vi "Read Both Fans Fault and State.vi"(8 "error in (no error)":cluster{"状态":bool, "代码":i32, "源":string} caption="错误输入（无错误）", 11 "双风扇输入":refnum<class "Dual Fan.lvclass">) -> (0 "error out":cluster{"状态":bool, "代码":i32, "源":string} caption="错误输出", 1 "风扇B故障":bool, 2 "风扇B状态":bool, 3 "风扇A故障":bool, 5 "风扇A状态":bool)   [LabVIEW 2015, in "Dual Fan.lvlib" / "Dual Fan.lvclass"]
doc: "子类中必须对该方法进行重写以读取两个风扇的信息：故障和状态（即风扇是否已打开）。"
uses:
  Dual Fan.lvclass
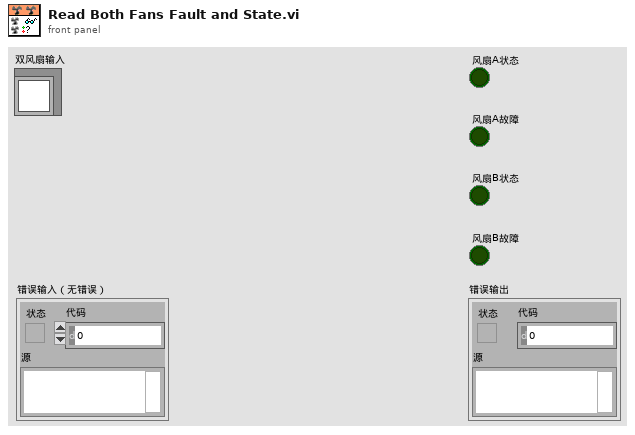
[diagram p1: front panel]
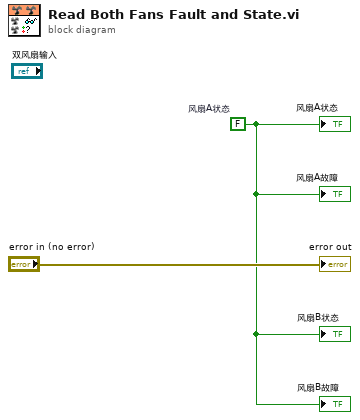
[diagram p0: block diagram]
diagram:
  w1 = FALSE  # 风扇A状态
  "风扇A故障" <- w1
  "error out" <- "error in (no error)"
  "风扇B故障" <- w1
  "风扇B状态" <- w1
  "风扇A状态" <- w1
